vi "Volt_AutoScalling_Osc_Dual_Channel_ControlvSUM.vi"(0 "VISA Oscilloscope":refnum<visa-resource-name>, 5 "Voltage In":dbl, 7 "Att":dbl, 9 "Clip":dbl=8.0, 11 "error in":errorcluster) -> (4 "VISA resource name out":refnum<visa-resource-name>, 15 "error out":errorcluster)   [LabVIEW 2012]
uses:
  <instrlib>/Agilent 8000 Series/Agilent 8000 Series.lvlib
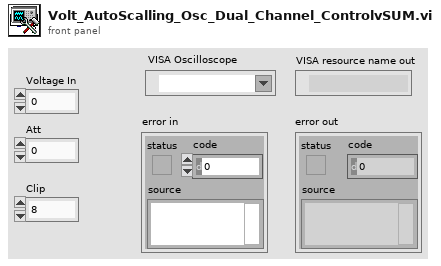
[diagram p1: front panel]
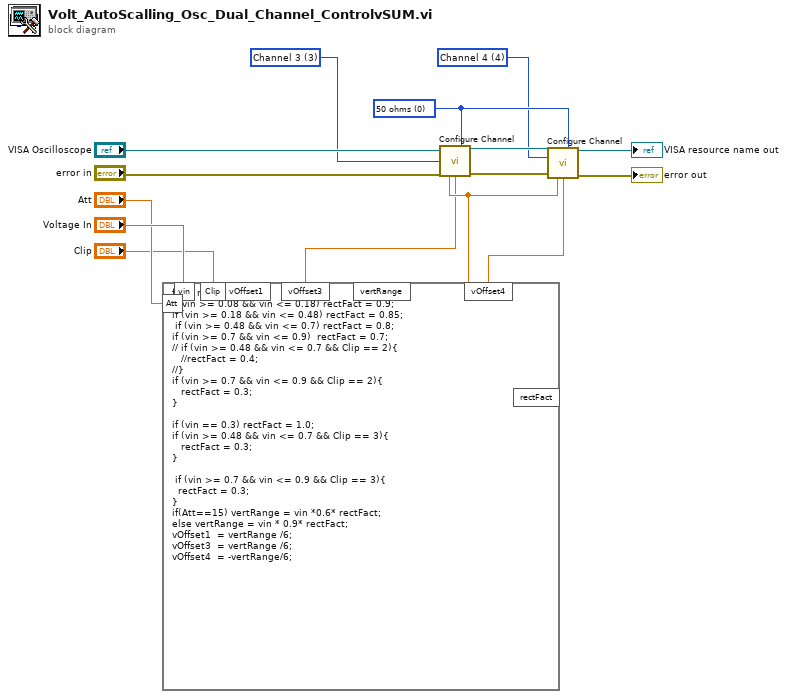
[diagram p0: block diagram]
diagram:
  w9 = 3 items=["Channel 1"=1, "Channel 2"=2, "Channel 3"=3, "Channel 4"=4] ("Channel (1: Channel 1)")
  w14 = u32 0 items=["50 ohms", "1 Mohms"] ("Input Impedance (1: 1 Mohms)")
  w13 = 4 items=["Channel 1"=1, "Channel 2"=2, "Channel 3"=3, "Channel 4"=4] ("Channel (1: Channel 1)")
  n1 = formula code="float rectFact = 1;\nif(vin >= 0.08 && vin <= 0.18) rectFact = 0.9;\nif (vin >= 0.18 && vin <= 0.48) rectFact = 0.85;\n if (vin >= 0.48 && vin <= 0.7) rectFact = 0.8;\nif (vin >= 0.7 && vin <= 0.9)  rectFact = 0.7;\n// if (vin >= 0.48 && vin <= 0.7 && Clip == 2){\n   //rectFact = 0.4;\n//}\nif (vin >= 0.7 && vin <= 0.9 && Clip == 2){\n   rectFact = 0.3;\n}\n\nif (vin == 0.3) rectFact = 1.0;\nif (vin >= 0.48 && vin <= 0.7 && Clip == 3){\n   rectFact = 0.3;\n}\n\n if (vin >= 0.7 && vin <= 0.9 && Clip == 3){\n  rectFact = 0.3;\n}\nif(Att==15) vertRange = vin *0.6* rectFact;\nelse vertRange = vin * 0.9* rectFact;\nvOffset1  = vertRange /6;\nvOffset3  = vertRange /6;\nvOffset4  = -vertRange/6;"("vin"="Voltage In", "Att"="Att", "Clip"="Clip") -> ("vOffset3"=w2:dbl, "vOffset4"=w1:dbl, "vertRange"=w5:dbl)  [unwired: 2 out]
  n2 = call <instrlib>:"Configure Channel.vi"("VISA resource name"="VISA Oscilloscope", "Input Impedance (1: 1 Mohms)"=w14, "Channel (1: Channel 1)"=w9, "error in (no error)"="error in", "Vertical Range (2.0 V)"=w5, "Vertical Offset (0.0 V)"=w2) -> ("VISA resource name out"=w15:refnum<visa-resource-name>, "error out"=w10:errorcluster)  [unwired: 8 in]
  n3 = call <instrlib>:"Configure Channel.vi"("VISA resource name"=w15, "Input Impedance (1: 1 Mohms)"=w14, "Channel (1: Channel 1)"=w13, "error in (no error)"=w10, "Vertical Range (2.0 V)"=w5, "Vertical Offset (0.0 V)"=w1) -> ("VISA resource name out"=→"VISA resource name out":refnum<visa-resource-name>, "error out"=→"error out":errorcluster)  [unwired: 8 in]
